vi "data aq.vi"() -> ()   [LabVIEW 2009]
uses:
  <vilib>/Utility/file.llb/Write To Spreadsheet File (string).vi
  <vilib>/Utility/file.llb/Read From Spreadsheet File (DBL).vi
panel:
  out "winning effort player 2":string[][](array[string])
  out "loosing effort player 1":string[][](array[string])
  out "loosing effort player 2":string[][](array[string])
  out "winning effort player 1":string[][](array[string])
  out "FULL GAME player 1":string[][](array[string])
  out "FULL GAME player 2":string[][](array[string])
  out "point 2 coded":dbl[][](array[numeric])
  out "point 1 coded":dbl[][](array[numeric])
  out "point 2 rally":dbl[](array[numeric])
  out "point 1 rally":dbl[](array[numeric])
  out "start/end":dbl[](array[numeric])
  out "point 2":dbl[](array[numeric])
  out "point 1":dbl[](array[numeric])
  out "all rows":dbl[][](array[numeric]) format="%0.3f"
  in  "Data file":path caption="Read data from file"
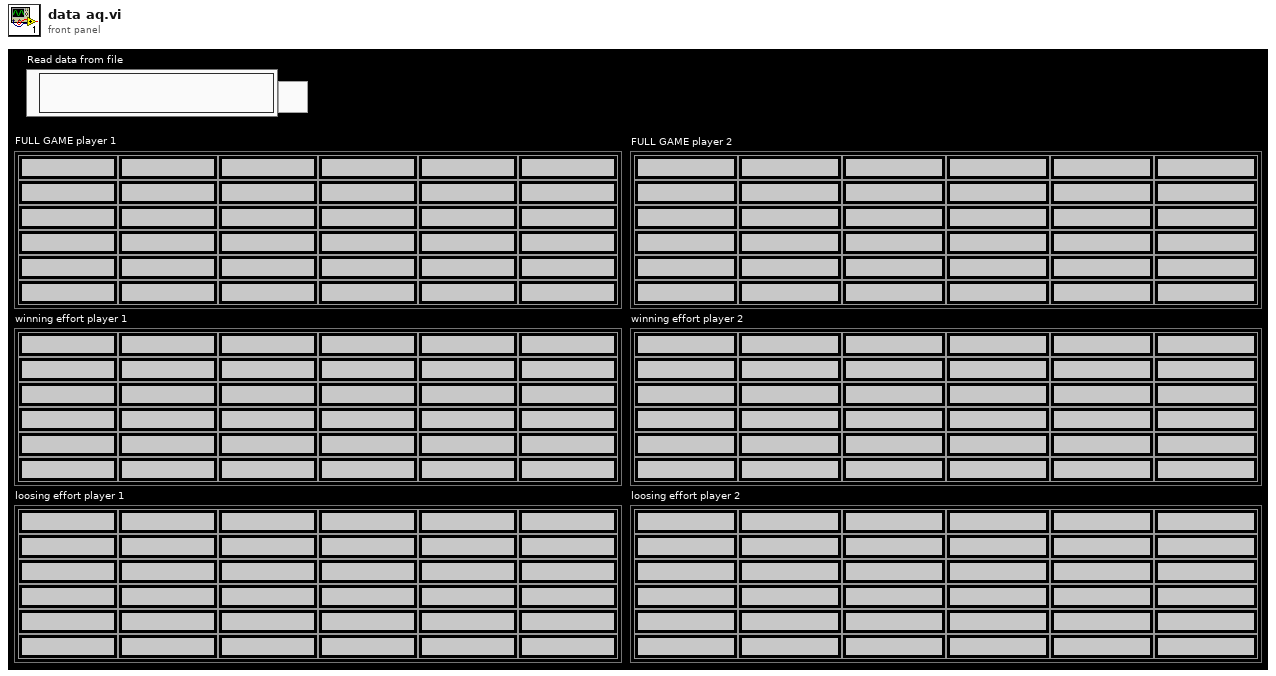
[diagram p1: front panel]
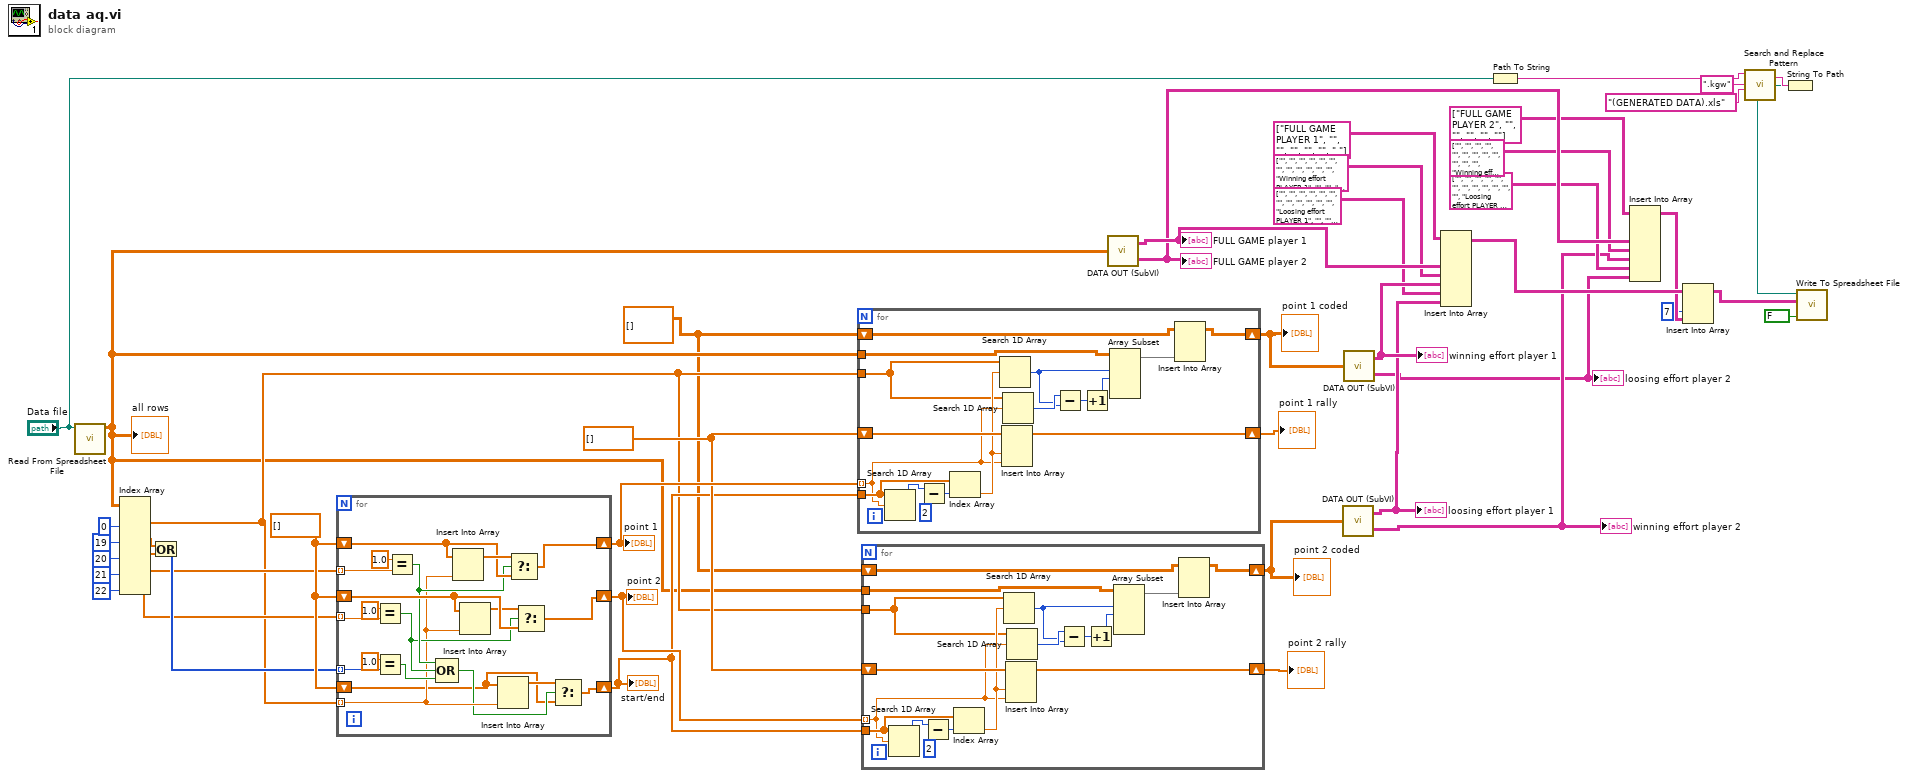
[diagram p0: block diagram]
diagram:
  w27 = dbl[][] [] ("subarray")
  w32 = dbl[] [] ("subarray")
  w38 = dbl[] [] ("subarray")
  n1 = call-poly <vilib>:"Read From Spreadsheet File.vi"("file path (dialog if empty)"="Data file") -> ("all rows"=w28:dbl[][])  [unwired: 6 in, 4 out]
  "all rows" <- w28
  n2 = Index Array(array=w28, index (col) #1=0 ("disabled index (col)"), index (col) #2=19 ("index (col)"), index (col) #3=20 ("index (col)"), index (col) #4=21 ("index (col)"), index (col) #5=22 ("index (col)")) -> (element #1=w29:dbl[], element #2=w40:dbl[], element #3=w39:dbl[], element #4=w36:dbl[], element #5=w35:dbl[])  [unwired: 5 in]
  n3 = Or(x=w40, y=w39) -> (x .or. y?=w37:i32[])
  n4 = for {
    tunnel: w36 -> [w65] mode=indexing
    tunnel: w29 -> [w49] mode=indexing
    tunnel: w37 -> [w54] mode=indexing
    tunnel: w35 -> [w59] mode=indexing
    shift-right: [w62] -> w34
    shift-left: w38 -> [w61]
    shift-right: [w56] -> w31
    shift-left: w38 -> [w58]
    shift-right: [w46] -> w30
    shift-left: w38 -> [w47]
    n5 = Equal?(x=1.0, y=w59) -> (x = y?=w52:bool)
    n6 = Equal?(x=1.0, y=w54) -> (x = y?=w51:bool)
    n7 = Equal?(x=1.0, y=w65) -> (x = y?=w53:bool)
    n8 = Compound Arithmetic op=OR(w53, w52, w51) -> (w48:bool)
    n9 = Insert Into Array(array=w61, new element=w49) -> (w63:dbl[])  [unwired: 1 in]
    n10 = Insert Into Array(array=w58, new element=w49) -> (w57:dbl[])  [unwired: 1 in]
    n11 = Insert Into Array(array=w47, new element=w49) -> (w50:dbl[])  [unwired: 1 in]
    n12 = Select(t=w63, s=w53, f=w61) -> (s? t:f=w62:dbl[])
    n13 = Select(t=w57, s=w52, f=w58) -> (s? t:f=w56:dbl[])
    n14 = Select(t=w50, s=w48, f=w47) -> (s? t:f=w46:dbl[])
  }
  "point 1" <- w34
  "point 2" <- w31
  "start/end" <- w30
  n15 = for {
    tunnel: w34 -> [w74] mode=indexing
    tunnel: w30 -> [w82]
    shift-right: [w79] -> w33
    shift-left: w32 -> [w80]
    tunnel: w28 -> [w72]
    tunnel: w29 -> [w75]
    shift-right: [w68] -> w25
    shift-left: w27 -> [w70]
    n16 = Search 1D Array(1D array=w82, element=w74) -> (index of element=w78:i32)  [unwired: 1 in]
    n17 = Subtract(x=w78, y=2) -> (x-y=w81:i32)
    n18 = Index Array(array=w82, index=w81) -> (element=w76:dbl)
    n19 = Search 1D Array(1D array=w75, element=w76) -> (index of element=w71:i32)  [unwired: 1 in]
    n20 = Insert Into Array(array=w80, new element #1=w76, new element #2=w74) -> (w79:dbl[])  [unwired: 1 in]
    n21 = Search 1D Array(1D array=w75, element=w74) -> (index of element=w73:i32)  [unwired: 1 in]
    n22 = Subtract(x=w73, y=w71) -> (x-y=w66:i32)
    n23 = Increment(x=w66) -> (x+1=w67:i32)
    n24 = Array Subset(array=w72, index (row)=w71, length (row)=w67) -> (w69:dbl[][])  [unwired: 2 in]
    n25 = Insert Into Array(array=w70, new element=w69) -> (w68:dbl[][])  [unwired: 2 in]
  }
  "point 1 rally" <- w33
  "point 1 coded" <- w25
  n26 = for {
    tunnel: w31 -> [w91] mode=indexing
    tunnel: w30 -> [w99]
    shift-right: [w96] -> w26
    shift-left: w32 -> [w97]
    tunnel: w28 -> [w89]
    tunnel: w29 -> [w92]
    shift-right: [w85] -> w24
    shift-left: w27 -> [w87]
    n27 = Search 1D Array(1D array=w99, element=w91) -> (index of element=w95:i32)  [unwired: 1 in]
    n28 = Subtract(x=w95, y=2) -> (x-y=w98:i32)
    n29 = Index Array(array=w99, index=w98) -> (element=w93:dbl)
    n30 = Search 1D Array(1D array=w92, element=w93) -> (index of element=w88:i32)  [unwired: 1 in]
    n31 = Insert Into Array(array=w97, new element #1=w93, new element #2=w91) -> (w96:dbl[])  [unwired: 1 in]
    n32 = Search 1D Array(1D array=w92, element=w91) -> (index of element=w90:i32)  [unwired: 1 in]
    n33 = Subtract(x=w90, y=w88) -> (x-y=w83:i32)
    n34 = Increment(x=w83) -> (x+1=w84:i32)
    n35 = Array Subset(array=w89, index (row)=w88, length (row)=w84) -> (w86:dbl[][])  [unwired: 2 in]
    n36 = Insert Into Array(array=w87, new element=w86) -> (w85:dbl[][])  [unwired: 2 in]
  }
  "point 2 rally" <- w26
  "point 2 coded" <- w24
  n37 = call "DATA OUT (SubVI).vi"("CODED DATA"=w28) -> ("FULL GAME player 1"=w22:string[][], "FULL GAME player 2"=w17:string[][])
  "FULL GAME player 2" <- w17
  "FULL GAME player 1" <- w22
  n38 = call "DATA OUT (SubVI).vi"("CODED DATA"=w24) -> ("FULL GAME player 1"=w18:string[][], "FULL GAME player 2"=w2:string[][])
  "winning effort player 2" <- w2
  "loosing effort player 1" <- w18
  n39 = call "DATA OUT (SubVI).vi"("CODED DATA"=w25) -> ("FULL GAME player 1"=w20:string[][], "FULL GAME player 2"=w1:string[][])
  "loosing effort player 2" <- w1
  "winning effort player 1" <- w20
  n40 = Insert Into Array(array=string[][] [["FULL GAME PLAYER 1", "", "", "", "", "", " "]], new element #1=w22, new element #2=string[][] [["", "", "", "", "", ""], ["", "", "", "", "", ""], ["Winning effort PLAYER 1", "", "", "", "", ""]], new element #3=w20, new element #4=string[][] [["", "", "", "", "", ""], ["", "", "", "", "", ""], ["Loosing effort PLAYER 1", "", "", "", "", ""]], new element #5=w18) -> (w13:string[][])  [unwired: 2 in]
  n41 = Path To String(path="Data file") -> (string=w7:string)
  n42 = Insert Into Array(array=string[][] [["FULL GAME PLAYER 2", "", "", "", "", ""]], new element #1=w17, new element #2=string[][] [["", "", "", "", "", ""], ["", "", "", "", "", ""], ["Winning effort PLAYER 2", "", "", "", "", ""]], new element #3=w2, new element #4=string[][] [["", "", "", "", "", ""], ["", "", "", "", "", ""], ["Loosing effort PLAYER 2", "", "", "", "", ""]], new element #5=w1) -> (w12:string[][])  [unwired: 2 in]
  n43 = Insert Into Array(array=w13, index (col)=7 ("disabled index (col)"), new element=w12) -> (w3:string[][])  [unwired: 1 in]
  n44 = call <vilib>:"Search and Replace Pattern.vi"("string"=w7, "regular expression (\"\")"=".kgw" ("regular expression (\"\")"), "replace string (\"\")"="(GENERATED DATA).xls" ("replace string (\"\")")) -> ("result string"=w6:string)  [unwired: 2 in, 1 out]
  n45 = String To Path(string=w6) -> (path=w4:path)
  n46 = call-poly <vilib>:"Write To Spreadsheet File.vi"("append to file? (new file:F)"=FALSE, "2D data"=w3, "file path (dialog if empty)"=w4) -> ()  [unwired: 5 in, 1 out]
